vi "rql_Update Fréquence.vi"(4 "Show in Debugger?":bool=TRUE, 6 "Message Priority":T1=enum."Normal", 8 "error in":errorcluster, 10 "Data in":T2={"max freq (50 ... 18 500)"=200} {"max freq (50 ... 18 500)" min=50 max=18500 step=1}, 11 "UI SmarAct in":refnum<class "UI SmarAct.lvclass">) -> (0 "error out":errorcluster, 3 "dup UI SmarAct out":refnum<class "UI SmarAct.lvclass">)   [LabVIEW 2024, in "UI SmarAct.lvclass"]
doc: "This VI sends a <b>Local API Request</b> message to an MHL case of the Worker that owns this VI.\n---\nMise à jour de la fréquence Max de la platine"
uses:
  UI SmarAct.lvclass
  C:/Program Files (x86)/National Instruments/LabVIEW 2024/vi.lib/addons/_Workers/Library/Classes/Worker/Worker.lvclass
  <vilib>/addons/_Workers/Library/Classes/Message/Priority.ctl
  <vilib>/addons/_Workers/Library/Case Label.ctl
  <vilib>/addons/_Workers/Library/Classes/Message Queue/Message Queue.lvclass
  <vilib>/addons/_Workers/Library/Workers.lvlib
  <vilib>/addons/_Workers/Library/Classes/Message/Message.lvclass
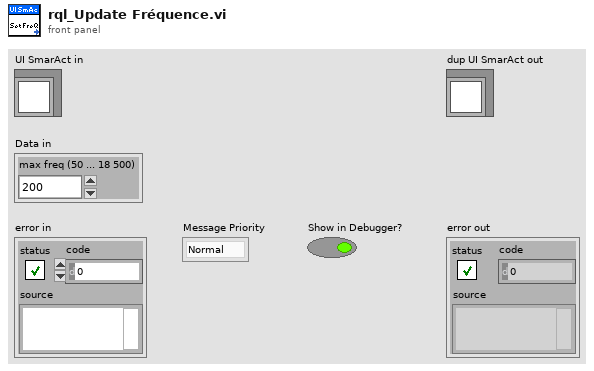
[diagram p1: front panel]
types:
  T1 = typedef "Workers.lvlib/Message.lvclass/Priority.ctl" = enum16{"Low", "Normal", "High"}
  T2 = typedef "UI SmarAct.lvclass/rql_Update Fréquence.ctl" = cluster{"max freq (50 ... 18 500)":u32}
  T3 = typedef "Workers.lvlib/Case Label.ctl" = string
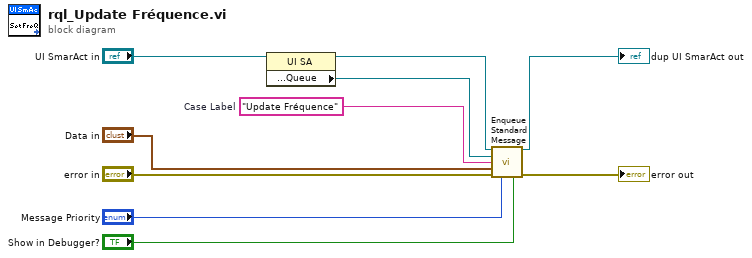
[diagram p0: block diagram]
diagram:
  w1 = T3 "Update Fréquence"  # Case Label
  n1 = property class="UI SA"(reference="UI SmarAct in") -> (reference out=w3:refnum<class "UI SmarAct.lvclass">, "Accessors:Read:Public API:Queue"=w2:refnum<class "Message Queue.lvclass">)  [unwired: 1 in, 1 out]
  n2 = call-dynamic "Enqueue Standard Message.vi"("Worker"=w3, "Message Queue"=w2, "Case Label"=w1, "Data"="Data in", "error in (no error)"="error in", "Priority (Normal)"="Message Priority", "Send Message to Debugger? (T)"="Show in Debugger?") -> ("dup Worker out"=→"dup UI SmarAct out":refnum<class "UI SmarAct.lvclass">, "error out"=→"error out":errorcluster)  [unwired: 7 in]
